vi "get_component_type_name.vi"(8 "error in (no error)":errorcluster, 11 "GenericSignalWriter in":refnum<class "GenericSignalWriter.lvclass">) -> (0 "error out":errorcluster, 2 "component type":string="SignalWriter", 3 "GenericSignalWriter out":refnum<class "GenericSignalWriter.lvclass">)   [LabVIEW 2010, in "GenericSignalWriter.lvclass"]
uses:
  GenericSignalWriter.lvclass
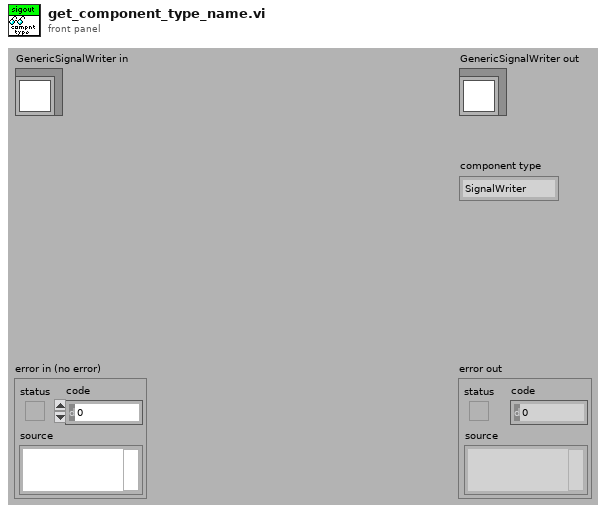
[diagram p1: front panel]
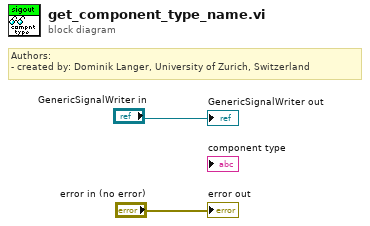
[diagram p0: block diagram]
diagram:
  # "Authors: \n- created by: Dominik Langer, University of Zurich, Switzerland"
  "error out" <- "error in (no error)"
  "GenericSignalWriter out" <- "GenericSignalWriter in"
